vi "myRIO_BRig_RT_dataCurrent_laser1_tCue1_start.vi"() -> (2 "output_laser1_tCue1_start":i32)   [LabVIEW 2014]
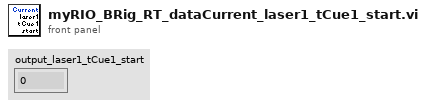
[diagram p1: front panel]
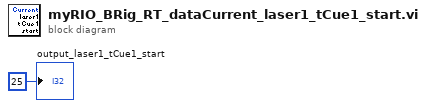
[diagram p0: block diagram]
diagram:
  "output_laser1_tCue1_start" <- 25 ("output_iBlock")
